vi "SetPower.vi"(8 "error in (no error)":errorcluster, 9 "Value":dbl format="%#_13g", 10 "Label":string, 11 "Laser_Oxxius in":refnum<class "Laser_Oxxius.lvclass">) -> (0 "error out":errorcluster, 3 "Laser_Oxxius out":refnum<class "Laser_Oxxius.lvclass">)   [LabVIEW 2020, in "Laser_Oxxius.lvlib" / "Laser_Oxxius.lvclass"]
uses:
  Laser_Oxxius.lvclass
  Laser_Oxxius.lvclass/Laser_Oxxius.ctl
  E:/Development/DevHardSoftware/MicroscopyFramework/Model/Hardware Layer/Real Hardware/Laser_Oxxius/Laser_Oxxius/Dependency/Oxxius_Boxx.dll
  Dependency/Oxxius_Boxx.dll
  Hardware Abstraction Layer/Component/Laser/Laser/Laser.lvclass
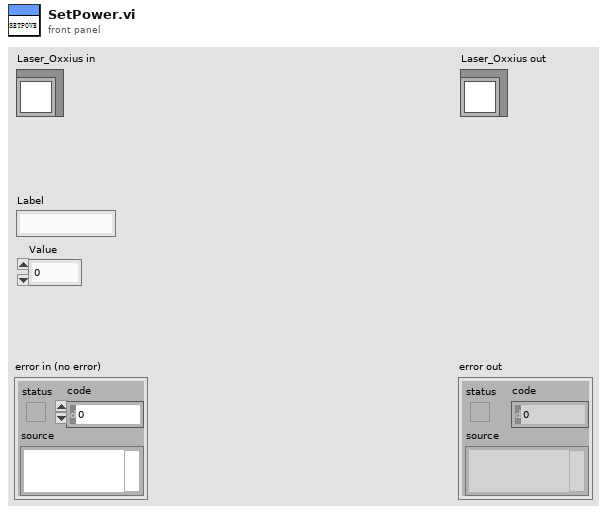
[diagram p1: front panel]
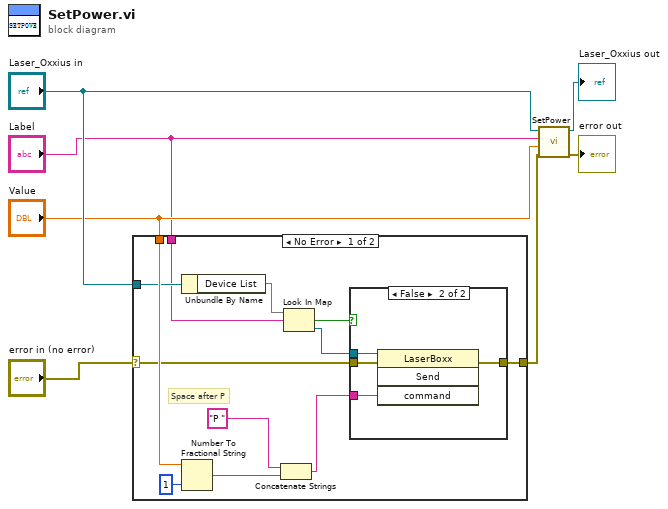
[diagram p0: block diagram]
diagram:
  n1 = case shown="No Error" "error in (no error)" {
    selector: "error in (no error)" -> [w15 w25]
    tunnel: "Laser_Oxxius in" -> [w14 _]
    tunnel: [w10 w25] -> w3
    tunnel: "Value" -> [w19 _]
    tunnel: "Label" -> [w12 _]
    frame No Error {
      # "Space after P"
      n2 = Unbundle By Name(w14) -> ("Device List"=w13:map{string, refnum<k24>})
      n3 = Number To Fractional String(number=w19, precision (6)=i16 1) -> (F-format string=w18:string)  [unwired: 2 in]
      n4 = Concatenate Strings("P " ("string"), w18) -> (w16:string)
      n5 = Look In Map(map=w13, key=w12) -> (key not found?=w9:bool, value=w11:refnum<k24>)  [unwired: 1 in]
      n6 = case shown="False" w9 {
        tunnel: w16 -> [_ w24]
        tunnel: w15 -> [w20 w23]
        tunnel: w11 -> [_ w22]
        tunnel: [w20 w21] -> w10
        frame True {
        }
        frame False {
          n7 = invoke class="LaserBoxx" method="Send"(reference=w22, error in=w23, "command"=w24) -> (error out=w21:errorcluster)  [unwired: 1 in, 3 out]
        }
      }
    }
    frame Error {
    }
  }
  n8 = call-parent "SetPower.vi"("error in (no error)"=w3, "Value"="Value", "Label"="Label", "Laser in"="Laser_Oxxius in") -> ("error out"=→"error out":errorcluster, "Laser out"=→"Laser_Oxxius out":refnum<class "Laser_Oxxius.lvclass">)  [unwired: 6 in]
